vi "Detector Get Image delete me.vi"(8 "error in (no error)":errorcluster, 11 "PRIME Detector in":refnum<class "PRIME Detector.lvclass">) -> (0 "error out":errorcluster, 1 "FITS Detector Settings":T1, 2 "Images":T2[](array[typedef]) {"Detector #" items=["None", "YJ", "HK"]}, 3 "PRIME Detector out":refnum<class "PRIME Detector.lvclass">, 4 "Message Log":string)   [LabVIEW 2020]
uses:
  PRIME Detector.lvclass
  C:/Development/prime/Prime-RIMAS/Detector/Detector Class/Detector Class.lvclass
  C:/Development/prime/Prime-RIMAS/Detector/Detector Class/PRIME Detector/PRIME Detector.lvclass
  Detector Image typedef cluster.ctl
  Detector Class.lvclass
  RIMAS Observation Config.ctl
panel:
  # "sec"
  # "sec"
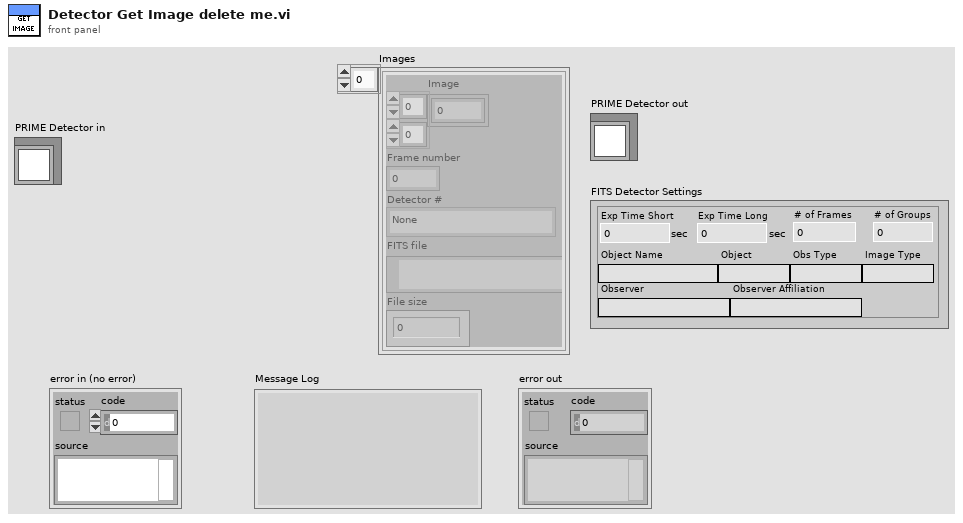
[diagram p1: front panel]
types:
  T1 = typedef "RIMAS Observation Config.ctl" = cluster{"Exp Time Short":dbl, "# of Frames":dbl, "Exp Time Long":dbl, "# of Groups":dbl, "Object Name":string, "Object":string, "Obs Type":string, "Image Type":string, "Observer":string, "Observer Affiliation":string}
  T2 = typedef "Detector Class.lvclass/Detector Image typedef cluster.ctl" = cluster{"Image":sgl[][], "Frame number":i32, "Detector #":u16, "FITS file":path, "File size":i64}
  T3 = typedef "PRIME Detector cluster Status.ctl" = cluster{"Cmd Start Time":timestamp, "Command":string, "Complete?":bool, "Cmd Complete Time":timestamp, "Exp Time Remaining":dbl, "Total Frames":i32, "Exp Frames":cluster{"CAMERA0":string[], "CAMERA1":string[], "CAMERA2":string[], "CAMERA3":string[]}, "Intermediate Frames":cluster{"CAMERA0":string[], "CAMERA1":string[], "CAMERA2":string[], "CAMERA3":string[]}, "Final Reduced Frame":cluster{"CAMERA0":string, "CAMERA1":string, "CAMERA2":string, "CAMERA3":string}}
  T4 = cluster{"CAMERA0":string[], "CAMERA1":string[], "CAMERA2":string[], "CAMERA3":string[]}
  T5 = cluster{"CAMERA0":string, "CAMERA1":string, "CAMERA2":string, "CAMERA3":string}
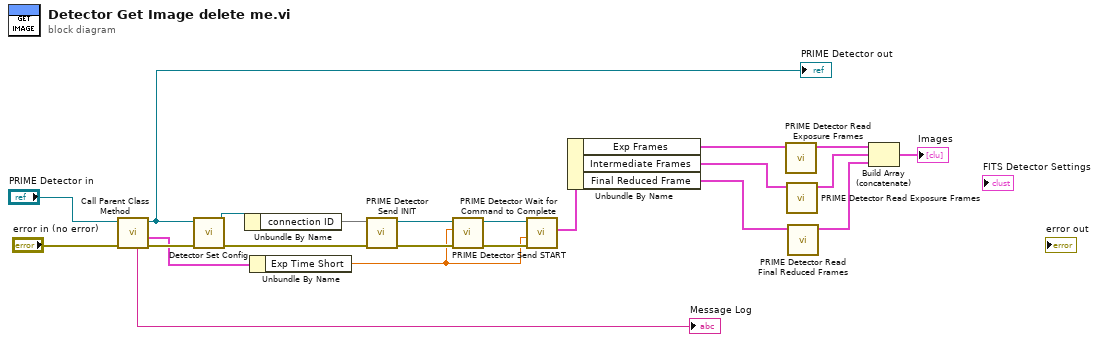
[diagram p0: block diagram]
diagram:
  n1 = call-parent "Call Parent Class Method"("error in (no error)"="error in (no error)", "Detector Class in"="PRIME Detector in") -> ("error out"=w18:errorcluster, "FITS Detector Settings"=w12:T1, "Detector Class out"=w15:refnum<class "PRIME Detector.lvclass">, "Message Log"=→"Message Log":string)  [unwired: 5 in, 1 out]
  "PRIME Detector out" <- w15
  n2 = call-dynamic "Detector Set Config.vi"("error in (no error)"=w18, "PRIME Detector in"=w15) -> ("error out"=w16:errorcluster, "PRIME Detector out"=w17:refnum<class "PRIME Detector.lvclass">)  [unwired: 8 in]
  n3 = Unbundle By Name(w17) -> ("connection ID"=w19)
  n4 = Unbundle By Name(w12) -> ("Exp Time Short"=w10:dbl)
  n5 = call "PRIME Detector Send INIT.vi"("error in (no error)"=w16, "connection ID"=w19) -> ("error out"=w13:errorcluster, "connection ID out"=w14:refnum<k5>)  [unwired: 8 in]
  n6 = call "PRIME Detector Send START.vi"("error in (no error)"=w13, "Exposure Time"=w10, "connection ID"=w14) -> ("error out"=w11:errorcluster, "connection ID out"=w9:refnum<k5>)  [unwired: 7 in]
  n7 = call "PRIME Detector Wait for Command to Complete.vi"("error in (no error)"=w11, "Exp Time"=w10, "connection ID"=w9) -> ("Status"=w8:T3)  [unwired: 6 in, 2 out]
  n8 = Unbundle By Name(w8) -> ("Exp Frames"=w7:T4, "Intermediate Frames"=w6:T4, "Final Reduced Frame"=w5:T5)
  n9 = call "PRIME Detector Read Exposure Frames.vi"("Exp Frames"=w7) -> ("Images"=w4:T2[])  [unwired: 10 in]
  n10 = call "PRIME Detector Read Exposure Frames.vi"("Exp Frames"=w6) -> ("Images"=w3:T2[])  [unwired: 10 in]
  n11 = call "PRIME Detector Read Final Reduced Frames.vi"("Final Reduced Frame"=w5) -> ("Images"=w2:T2[])  [unwired: 10 in]
  n12 = Build Array (concatenate)(w4, w3, w2) -> (→"Images":T2[])
